vi "staticUpdateHWError.vi"(8 "error in (no error)":errorcluster, 11 "AtomChipHWC in":refnum<class "AtomChipHWC.lvclass">) -> (0 "error out":errorcluster, 3 "AtomChipHWC out":refnum<class "AtomChipHWC.lvclass">)   [LabVIEW 2009, in "Hardware.lvlib" / "HWControllers.lvlib" / "AtomChipHWC.lvclass"]
uses:
  AtomChipHWC.lvclass
  AtomChipHWC.lvclass/AtomChipHWC.ctl
  Channels/Digital/DigitalOutput.lvclass
  Channels/VoltOutput/AnalogOutput.lvclass
  Channels/DDSOutput/Generic/DDSOutput.lvclass
  Network Controllers/CameraNetworkController/CameraNetworkController.lvclass
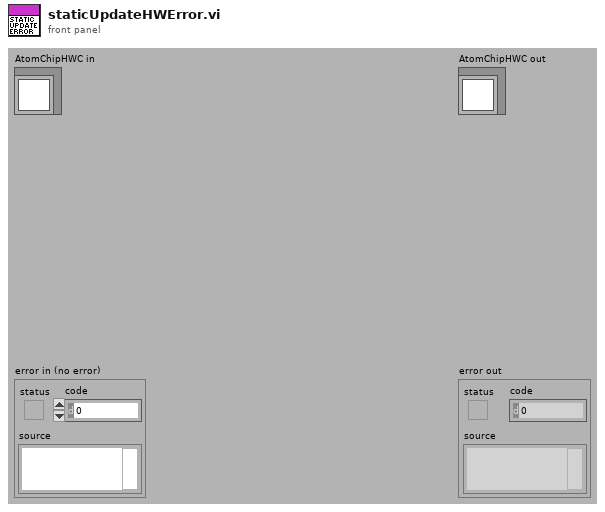
[diagram p1: front panel]
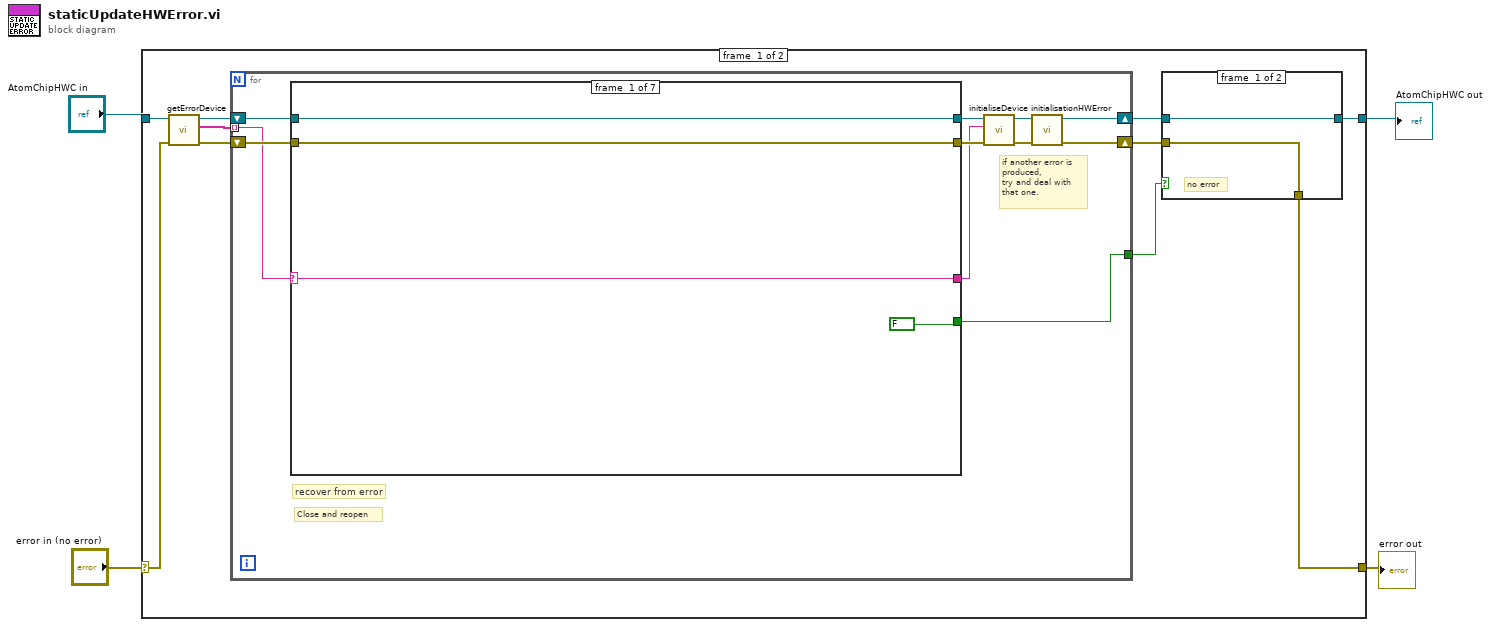
[diagram p0: block diagram]
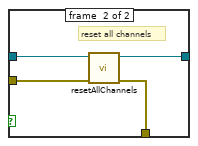
[diagram p2: hidden frame]
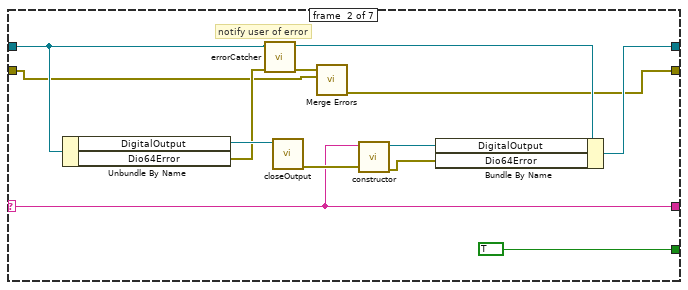
[diagram p3: hidden frame]
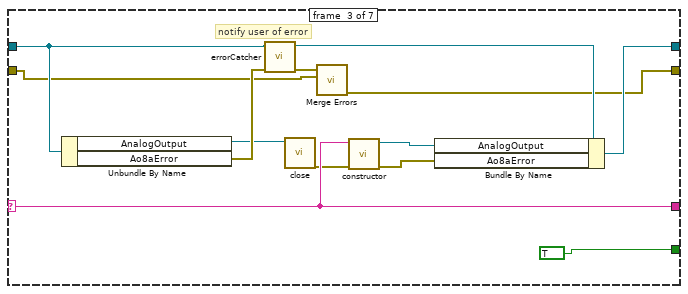
[diagram p4: hidden frame]
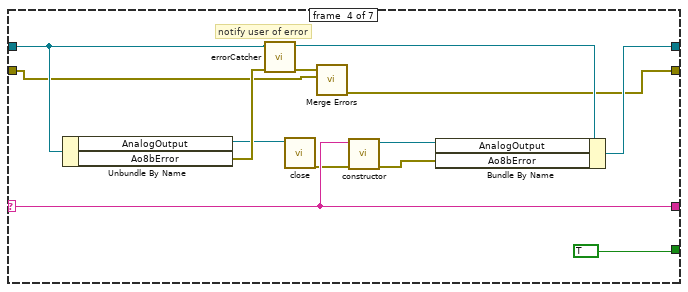
[diagram p5: hidden frame]
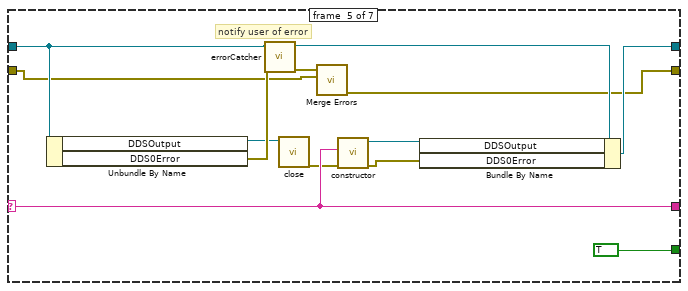
[diagram p6: hidden frame]
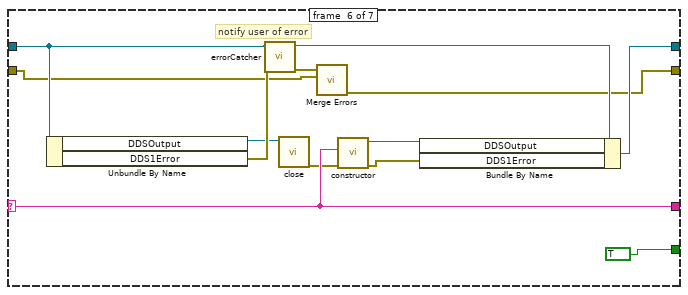
[diagram p7: hidden frame]
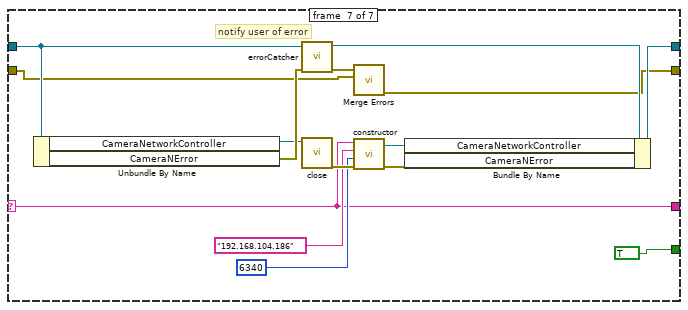
[diagram p8: hidden frame]
diagram:
  n1 = case shown="No Error" "error in (no error)" {
    selector: "error in (no error)" -> [w13 w116]
    tunnel: "AtomChipHWC in" -> [w14 w117]
    tunnel: [w7 w117] -> w2
    tunnel: [w6 w116] -> w1
    frame #0 {
      n2 = call "getErrorDevice.vi"("error in (no error)"=w13, "AtomChipHWC in"=w14) -> ("error out"=w10:errorcluster, "Devices"=w11:string[], "AtomChipHWC out"=w12:refnum<class "AtomChipHWC.lvclass">)  [unwired: 7 in]
      n3 = for {
        tunnel: w11 -> [w29] mode=indexing
        shift-right: [w23] -> w9
        shift-left: w12 -> [w31]
        shift-right: [w22] -> w8
        shift-left: w10 -> [w30]
        tunnel: [w21] -> w5
        # "Close and reopen"
        # "if another error is\nproduced,\ntry and deal with\nthat one."
        # "recover from error"
        n4 = case shown="Default" w29 {
          selector: w29 -> [w33 w37 w53 w66 w77 w90 w102]
          tunnel: w31 -> [w35 w44 w61 w74 w87 w100 w115]
          tunnel: [w35 w39 w56 w69 w82 w95 w110] -> w26
          tunnel: [w34 w38 w55 w68 w81 w94 w109] -> w25
          tunnel: w30 -> [w34 w40 w57 w70 w83 w96 w111]
          tunnel: [w33 w37 w53 w66 w77 w90 w102] -> w24
          tunnel: [FALSE TRUE TRUE TRUE TRUE TRUE TRUE] -> w21
          frame #0 {
          }
          frame #1 {
            # "notify user of error"
            n5 = Unbundle By Name(w44) -> ("DigitalOutput"=w48:refnum<class "DigitalOutput.lvclass">, "Dio64Error"=w42:errorcluster)
            n6 = call-dynamic "errorCatcher.vi"("error in (no error)"=w42, "HWController in"=w44) -> ("error out"=w41:errorcluster, "HWController out"=w43:refnum<class "AtomChipHWC.lvclass">)  [unwired: 8 in]
            n7 = call-dynamic "closeOutput.vi"("DigitalOutput in"=w48) -> ("error out"=w47:errorcluster)  [unwired: 10 in]
            n8 = call <vilib>:"Merge Errors.vi"("error in 2 (no error)"=w40, "error in 1 (no error)"=w41) -> ("error out"=w38:errorcluster)  [unwired: 5 in]
            n9 = call "constructor.vi"("error in (no error)"=w47, "deviceName"=w37) -> ("error out"=w45:errorcluster, "DigitalOutput out"=w46:refnum<class "DigitalOutput.lvclass">)  [unwired: 8 in]
            n10 = Bundle By Name(cluster=w43, "DigitalOutput"=w46, "Dio64Error"=w45) -> (w39:refnum<class "AtomChipHWC.lvclass">)
          }
          frame #2 {
            # "notify user of error"
            n11 = Unbundle By Name(w61) -> ("AnalogOutput"=w54:refnum<class "AnalogOutput.lvclass">, "Ao8aError"=w59:errorcluster)
            n12 = call-dynamic "errorCatcher.vi"("error in (no error)"=w59, "HWController in"=w61) -> ("error out"=w58:errorcluster, "HWController out"=w60:refnum<class "AtomChipHWC.lvclass">)  [unwired: 8 in]
            n13 = call-dynamic "close.vi"("AnalogOutput in"=w54) -> ("error out"=w52:errorcluster)  [unwired: 10 in]
            n14 = call <vilib>:"Merge Errors.vi"("error in 2 (no error)"=w57, "error in 1 (no error)"=w58) -> ("error out"=w55:errorcluster)  [unwired: 5 in]
            n15 = call "constructor.vi"("error in (no error)"=w52, "deviceName"=w53) -> ("error out"=w50:errorcluster, "AnalogOutput out"=w51:refnum<class "AnalogOutput.lvclass">)  [unwired: 8 in]
            n16 = Bundle By Name(cluster=w60, "AnalogOutput"=w51, "Ao8aError"=w50) -> (w56:refnum<class "AtomChipHWC.lvclass">)
          }
          frame #3 {
            # "notify user of error"
            n17 = Unbundle By Name(w74) -> ("AnalogOutput"=w67:refnum<class "AnalogOutput.lvclass">, "Ao8bError"=w72:errorcluster)
            n18 = call-dynamic "errorCatcher.vi"("error in (no error)"=w72, "HWController in"=w74) -> ("error out"=w71:errorcluster, "HWController out"=w73:refnum<class "AtomChipHWC.lvclass">)  [unwired: 8 in]
            n19 = call-dynamic "close.vi"("AnalogOutput in"=w67) -> ("error out"=w65:errorcluster)  [unwired: 10 in]
            n20 = call <vilib>:"Merge Errors.vi"("error in 2 (no error)"=w70, "error in 1 (no error)"=w71) -> ("error out"=w68:errorcluster)  [unwired: 5 in]
            n21 = call "constructor.vi"("error in (no error)"=w65, "deviceName"=w66) -> ("error out"=w63:errorcluster, "AnalogOutput out"=w64:refnum<class "AnalogOutput.lvclass">)  [unwired: 8 in]
            n22 = Bundle By Name(cluster=w73, "AnalogOutput"=w64, "Ao8bError"=w63) -> (w69:refnum<class "AtomChipHWC.lvclass">)
          }
          frame #4 {
            # "notify user of error"
            n23 = Unbundle By Name(w87) -> ("DDSOutput"=w80:refnum<class "DDSOutput.lvclass">, "DDS0Error"=w85:errorcluster)
            n24 = call-dynamic "errorCatcher.vi"("error in (no error)"=w85, "HWController in"=w87) -> ("error out"=w84:errorcluster, "HWController out"=w86:refnum<class "AtomChipHWC.lvclass">)  [unwired: 8 in]
            n25 = call-dynamic "close.vi"("DDSOutput in"=w80) -> ("error out"=w76:errorcluster)  [unwired: 10 in]
            n26 = call <vilib>:"Merge Errors.vi"("error in 2 (no error)"=w83, "error in 1 (no error)"=w84) -> ("error out"=w81:errorcluster)  [unwired: 5 in]
            n27 = call "constructor.vi"("error in (no error)"=w76, "device"=w77) -> ("error out"=w78:errorcluster, "DDSOutput out"=w79:refnum<class "DDSOutput.lvclass">)  [unwired: 8 in]
            n28 = Bundle By Name(cluster=w86, "DDSOutput"=w79, "DDS0Error"=w78) -> (w82:refnum<class "AtomChipHWC.lvclass">)
          }
          frame #5 {
            # "notify user of error"
            n29 = Unbundle By Name(w100) -> ("DDSOutput"=w93:refnum<class "DDSOutput.lvclass">, "DDS1Error"=w98:errorcluster)
            n30 = call-dynamic "errorCatcher.vi"("error in (no error)"=w98, "HWController in"=w100) -> ("error out"=w97:errorcluster, "HWController out"=w99:refnum<class "AtomChipHWC.lvclass">)  [unwired: 8 in]
            n31 = call-dynamic "close.vi"("DDSOutput in"=w93) -> ("error out"=w89:errorcluster)  [unwired: 10 in]
            n32 = call <vilib>:"Merge Errors.vi"("error in 2 (no error)"=w96, "error in 1 (no error)"=w97) -> ("error out"=w94:errorcluster)  [unwired: 5 in]
            n33 = call "constructor.vi"("error in (no error)"=w89, "device"=w90) -> ("error out"=w91:errorcluster, "DDSOutput out"=w92:refnum<class "DDSOutput.lvclass">)  [unwired: 8 in]
            n34 = Bundle By Name(cluster=w99, "DDSOutput"=w92, "DDS1Error"=w91) -> (w95:refnum<class "AtomChipHWC.lvclass">)
          }
          frame #6 {
            # "notify user of error"
            n35 = Unbundle By Name(w115) -> ("CameraNetworkController"=w108:refnum<class "CameraNetworkController.lvclass">, "CameraNError"=w113:errorcluster)
            n36 = call-dynamic "errorCatcher.vi"("error in (no error)"=w113, "HWController in"=w115) -> ("error out"=w112:errorcluster, "HWController out"=w114:refnum<class "AtomChipHWC.lvclass">)  [unwired: 8 in]
            n37 = call "close.vi"("CameraNetworkController in"=w108) -> ("error out"=w105:errorcluster)  [unwired: 9 in, 1 out]
            n38 = call <vilib>:"Merge Errors.vi"("error in 2 (no error)"=w111, "error in 1 (no error)"=w112) -> ("error out"=w109:errorcluster)  [unwired: 5 in]
            n39 = call "constructor.vi"("error in (no error)"=w105, "remote port"=u16 6340, "remote address"="192.168.104.186", "camera"=w102) -> ("error out"=w106:errorcluster, "CameraNetworkController out"=w107:refnum<class "CameraNetworkController.lvclass">)  [unwired: 6 in]
            n40 = Bundle By Name(cluster=w114, "CameraNetworkController"=w107, "CameraNError"=w106) -> (w110:refnum<class "AtomChipHWC.lvclass">)
          }
        }
        n41 = call "initialiseDevice.vi"("error in (no error)"=w25, "deviceName"=w24, "AtomChipHWC in"=w26) -> ("error out"=w27:errorcluster, "AtomChipHWC out"=w28:refnum<class "AtomChipHWC.lvclass">)  [unwired: 7 in]
        n42 = call-dynamic "initialisationHWError.vi"("error in (no error)"=w27, "AtomChipHWC in"=w28) -> ("error out"=w22:errorcluster, "AtomChipHWC out"=w23:refnum<class "AtomChipHWC.lvclass">)  [unwired: 8 in]
      }
      n43 = case shown="False" w5 {
        tunnel: w9 -> [w16 w20]
        tunnel: w8 -> [w15 w19]
        tunnel: [w16 w18] -> w7
        tunnel: [w15 w17] -> w6
        frame #0 {
          # "no error"
        }
        frame #1 {
          # "reset all channels"
          n44 = call-dynamic "resetAllChannels.vi"("error in (no error)"=w19, "AtomChipHWC in"=w20) -> ("error out"=w17:errorcluster, "AtomChipHWC out"=w18:refnum<class "AtomChipHWC.lvclass">)  [unwired: 8 in]
        }
      }
    }
    frame #1 {
    }
  }
  "error out" <- w1
  "AtomChipHWC out" <- w2
